vi "CRYReport Part ObjectMoved Event Callback.vi"(4 "TXTextControl":refnum<k7>, 5 "Event Data":cluster{"ObjectId":i16}, 6 "Control Ref":refnum<k7>, 7 "Event Common Data":T1) -> ()   [LabVIEW 2013]
uses:
  CRYReport Global.vi
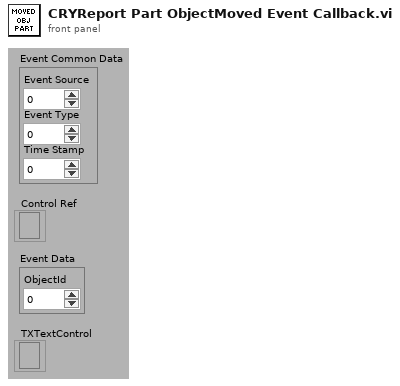
[diagram p1: front panel]
types:
  T1 = cluster{"Event Source":i32, "Event Type":u32, "Time Stamp":u32}
  T2 = cluster{"nID":i16, "sName":string, "pVIRef":refnum<vi>, "pSPRef":refnum<vi>, "sTitle":string, "nIDObject":i16, "nIDV":i16, "nWidth":i16, "nHeight":i16, "bImgChange":bool, "sType":string, "sState":string, "sPosition":string, "sData":string}
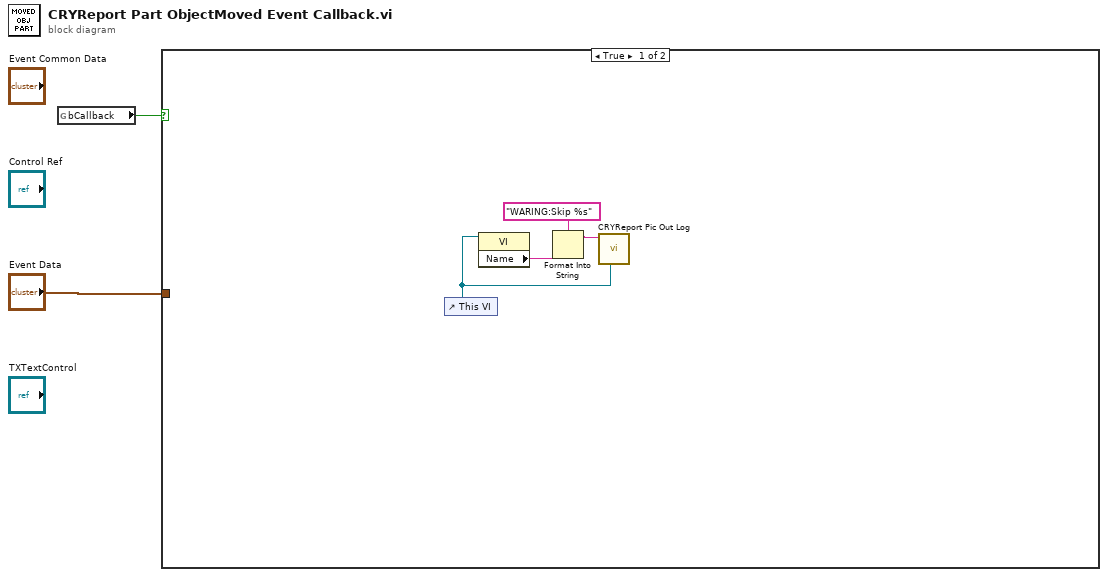
[diagram p0: block diagram]
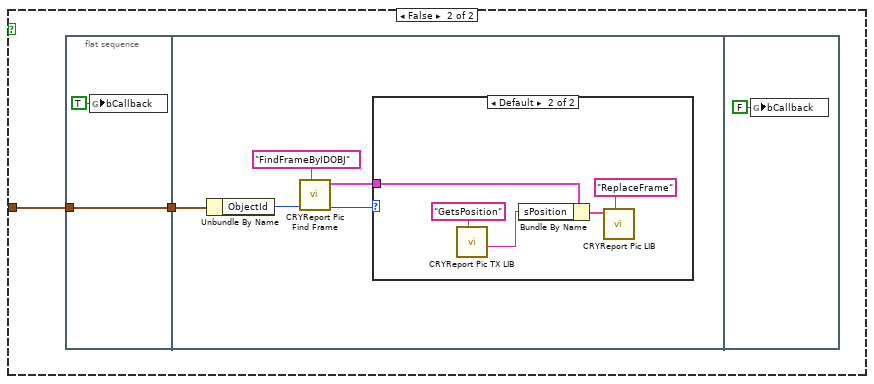
[diagram p2: hidden frame]
diagram:
  n1 = global read "CRYReport Global.vi" "bCallback"() -> (w1:bool)
  n2 = case shown="True" w1 {
    tunnel: "Event Data" -> [_ w7]
    frame True {
      n3 = control-ref of="This VI"() -> (w6:refnum<vi>)
      n4 = property class="VI"(reference=w6) -> ("Name"=w5:string)  [unwired: 1 in, 2 out]
      n5 = Format Into String(format string="WARING:Skip %s" ("string"), w5) -> (resulting string=w3:string)  [unwired: 2 in, 1 out]
      n6 = call "CRYReport Pic Out Log.vi"("vi reference"=w6, "sData"=w3) -> ()  [unwired: 10 in]
    }
    frame False {
      n7 = flat-sequence {
        tunnel: w7 -> [w10]
        tunnel: [w10] -> w8
        tunnel: w8 -> [w11]
        frame #0 {
          n8 = global write "CRYReport Global.vi" "bCallback"(TRUE ("bCallback")) -> ()
        }
        frame #1 {
          n9 = Unbundle By Name(w11) -> ("ObjectId"=w14:i16)
          n10 = call "CRYReport Pic Find Frame.vi"("sAction"="FindFrameByIDOBJ", "nData"=w14) -> ("nData_Out"=w13:i32, "cFrame_Out"=w12:T2)  [unwired: 8 in]
          n11 = case shown="Default" w13 {
            tunnel: w12 -> [_ w19]
            frame -1 {
            }
            frame Default {
              n12 = call "CRYReport Pic TX LIB.vi"("sAction"="GetsPosition") -> ("sData_Out"=w18:string)  [unwired: 8 in, 2 out]
              n13 = Bundle By Name(cluster=w19, "sPosition"=w18) -> (w17:T2)
              n14 = call "CRYReport Pic LIB.vi"("sAction"="ReplaceFrame", "cFrame"=w17) -> ()  [unwired: 6 in, 4 out]
            }
          }
        }
        frame #2 {
          n15 = global write "CRYReport Global.vi" "bCallback"(FALSE ("bCallback")) -> ()
        }
      }
    }
  }
